vi "Property Node (Filter).vi"   [LabVIEW 2017, in "nisyscfg.lvlib"]
doc: "Gets (reads) and/or sets (writes) properties for a user-defined filter. Wire the Save Changes VI to the property node after you have finished setting all the properties.\n\nRefer to Property Node (Filter) Descriptions for descriptions of the available properties."
uses:
  <vilib>/nisyscfg/nisyscfg.lvlib
  <resource>/objmgr/nisysapi.rc
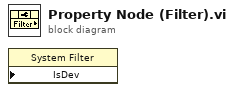
[diagram p0: block diagram]
diagram:
  n1 = property class="System Filter" props=["IsDev"]() -> ()  [unwired: 3 in, 2 out]
